vi "current source.vi"(6 "Settling time":dbl=1.0, 7 "Enable Output (T: Enable)":bool, 8 "error in (no error)":errorcluster, 10 "Output Level (0)":dbl, 11 "VISA current":refnum<visa-resource-name>="K2401") -> (0 "error out":errorcluster, 1 "Voltage":sgl format="%#_6e", 2 "Current":sgl, 3 "VISA resource name out":refnum<visa-resource-name>)   [LabVIEW 2019]
uses:
  <instrlib>/Keithley 24XX/Keithley 24XX.lvlib
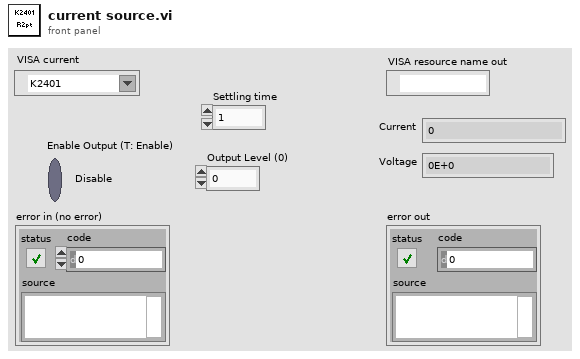
[diagram p1: front panel]
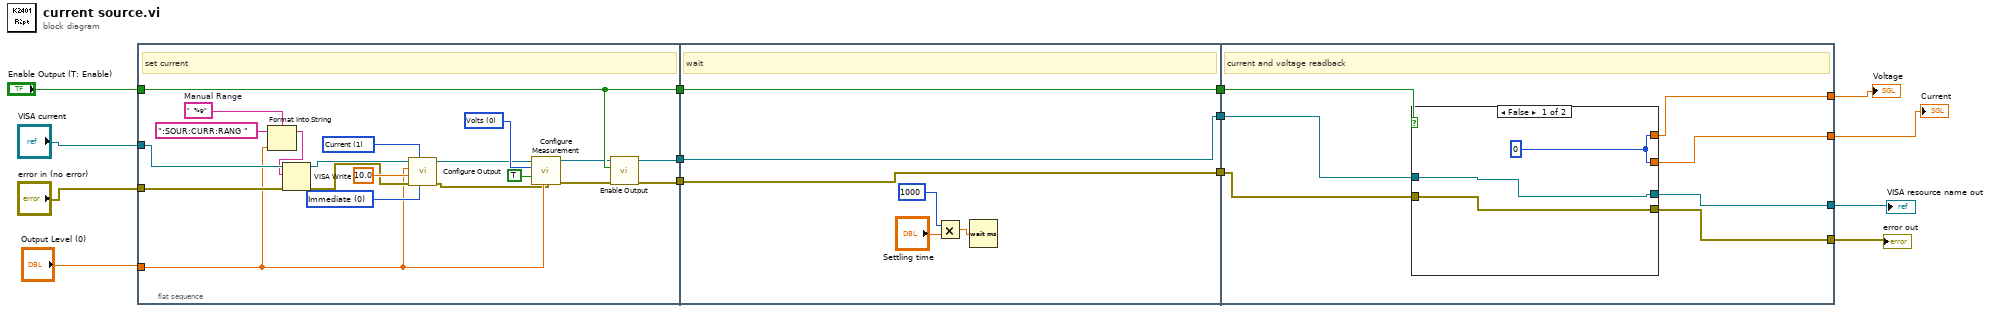
[diagram p0: block diagram]
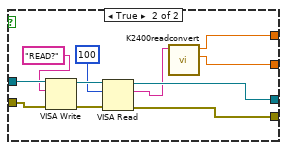
[diagram p2: hidden frame]
diagram:
  n1 = flat-sequence {
    tunnel: "VISA current" -> [w27]
    tunnel: "error in (no error)" -> [w26]
    tunnel: "Output Level (0)" -> [w22]
    tunnel: "Enable Output (T: Enable)" -> [w17]
    tunnel: [w17] -> w8
    tunnel: [w19] -> w7
    tunnel: [w18] -> w6
    tunnel: w8 -> [w37]
    tunnel: [w37] -> w5
    tunnel: w7 -> [w36]
    tunnel: w6 -> [w35]
    tunnel: [w36] -> w4
    tunnel: [w35] -> w3
    tunnel: [w41] -> w11
    tunnel: [w45] -> w10
    tunnel: [w44] -> w1
    tunnel: [w42] -> w2
    tunnel: w5 -> [w43]
    tunnel: w4 -> [w47]
    tunnel: w3 -> [w46]
    frame #0 {
      w29 = "  %g"  # Manual Range
      w31 = u16 0 items=["Volts", "Current", "Resistance"] ("Function (0: Volts)")
      w33 = u16 0 items=["Immediate", "Triggered"] ("Output Type  (0: Immediate)")
      w34 = u16 1 items=["Voltage", "Current"] ("Source Mode  (0: Voltage)")
      # "set current"
      n2 = Format Into String(format string=w29, initial string=":SOUR:CURR:RANG " ("Manual Range"), w22) -> (resulting string=w25:string)  [unwired: 1 in, 1 out]
      n3 = VISA Write(VISA resource name=w27, write buffer=w25, error in (no error)=w26) -> (VISA resource name out=w24:refnum<visa-resource-name>, error out=w23:errorcluster)  [unwired: 1 out]
      n4 = call <instrlib>:"Configure Output.vi"("Output Type  (0: Immediate)"=w33, "Source Mode  (0: Voltage)"=w34, "error in (no error)"=w23, "Compliance  Level (0.1)"=10.0, "Output Level (0)"=w22, "VISA resource name"=w24) -> ("error out"=w20:errorcluster, "VISA resource name out"=w21:refnum<visa-resource-name>)  [unwired: 4 in]
      n5 = call <instrlib>:"Configure Measurement.vi"("Manual Range (1.0)"=w22, "error in (no error)"=w20, "Enable Auto Range (T:Enable)"=TRUE, "Function (0: Volts)"=w31, "VISA resource name"=w21) -> ("error out"=w15:errorcluster, "VISA resource name out"=w16:refnum<visa-resource-name>)  [unwired: 5 in]
      n6 = call <instrlib>:"Enable Output.vi"("error in (no error)"=w15, "Enable Output (T: Enable)"=w17, "VISA resource name"=w16) -> ("error out"=w18:errorcluster, "VISA resource name out"=w19:refnum<visa-resource-name>)  [unwired: 7 in]
    }
    frame #1 {
      # "wait"
      n7 = Multiply(x=u32 1000, y="Settling time") -> (x*y=w39:dbl)
      n8 = Wait (ms)(milliseconds to wait=w39) -> ()  [unwired: 1 out]
    }
    frame #2 {
      # "current and voltage readback"
      n9 = case shown="False" w43 {
        tunnel: w47 -> [w49 w61]
        tunnel: w46 -> [w50 w60]
        tunnel: [w50 w56] -> w45
        tunnel: [w48 w51] -> w44
        tunnel: [w48 w52] -> w42
        tunnel: [w49 w55] -> w41
        frame False {
          w48 = 0
        }
        frame True {
          n10 = VISA Write(VISA resource name=w61, write buffer="READ?", error in (no error)=w60) -> (VISA resource name out=w57:refnum<visa-resource-name>, error out=w58:errorcluster)  [unwired: 1 out]
          n11 = VISA Read(VISA resource name=w57, byte count=u32 100, error in (no error)=w58) -> (VISA resource name out=w55:refnum<visa-resource-name>, read buffer=w53:string, error out=w56:errorcluster)  [unwired: 1 out]
          n12 = call "K2400readconvert.vi"("String"=w53) -> ("current"=w51:dbl, "voltage"=w52:dbl)  [unwired: 9 in]
        }
      }
    }
  }
  "Current" <- w1
  "VISA resource name out" <- w11
  "error out" <- w10
  "Voltage" <- w2
